vi "Read Shared Variables - SuNLaMP AO v2.vi"(9 "channel errors in (no errors)":errorcluster[](array[cluster])) -> (1 "channel errors out":errorcluster[](array[cluster]), 2 "data":dbl[](array[numeric]), 3 "UUIDs":string[](array[string])=["Flow Rate [g/s]", "Density [g/cm^3]", "Return Filter dP [psid]", "Outlet Filter and Flowmeter dp [psid]", "Cooler dP [psid]", "Cooler CO2 In [F]", "Cooler CO2 Out [F]", "Pump Frequency [%]", "Recirc Valve Open [%]"])   [LabVIEW 2020]
uses:
  <vilib>/ErrorRing/Error Ring.xnode
  <vilib>/Utility/error.llb/Error Cluster From Error Code.vi
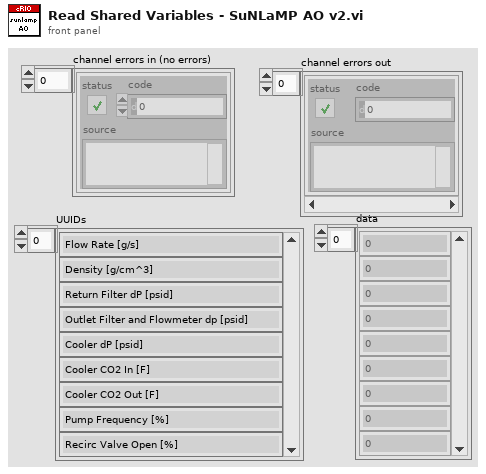
[diagram p1: front panel]
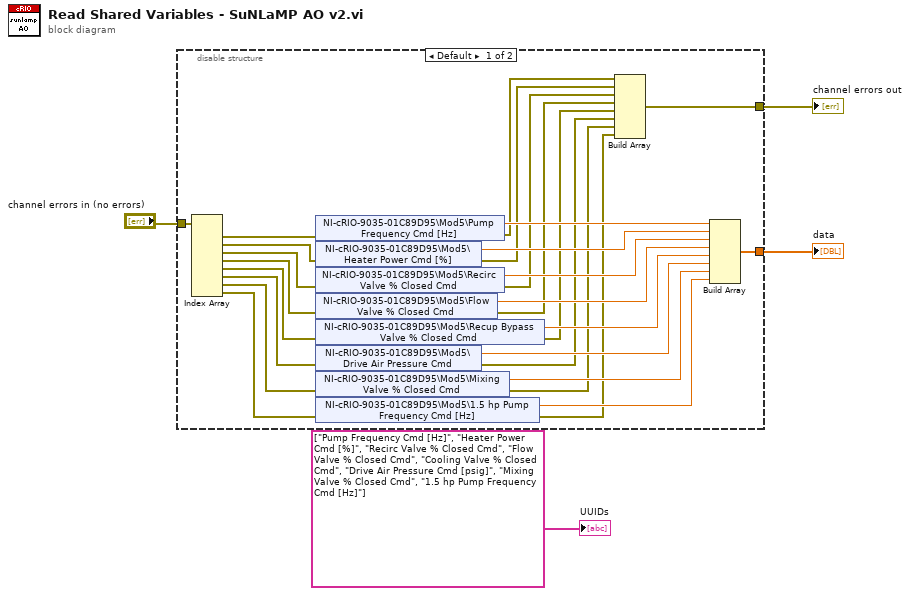
[diagram p0: block diagram]
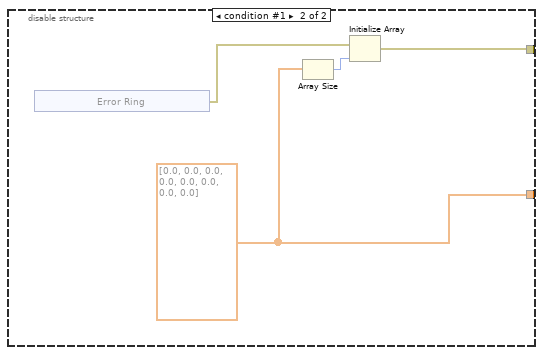
[diagram p2: hidden frame]
diagram:
  n1 = disable-structure shown="Default" {
    disable-tunnel: [w31 w34] -> w4
    disable-tunnel: [w30 w32] -> w2
    disable-tunnel: "channel errors in (no errors)" -> [w29 _]
    frame condition #0 (active) {
      n2 = Index Array(array=w29) -> (element #1=w12:errorcluster, element #2=w11:errorcluster, element #3=w10:errorcluster, element #4=w9:errorcluster, element #5=w8:errorcluster, element #6=w7:errorcluster, element #7=w6:errorcluster, element #8=w5:errorcluster)  [unwired: 8 in]
      n3 = shared-variable "NI-cRIO-9035-01C89D95\\Mod5\\Pump Frequency Cmd [Hz]"(error in=w12) -> (w21:dbl, error out=w13:errorcluster)
      n4 = shared-variable "NI-cRIO-9035-01C89D95\\Mod5\\Heater Power Cmd [%]"(error in=w11) -> (w22:dbl, error out=w14:errorcluster)
      n5 = shared-variable "NI-cRIO-9035-01C89D95\\Mod5\\Recirc Valve % Closed Cmd"(error in=w10) -> (w23:dbl, error out=w15:errorcluster)
      n6 = shared-variable "NI-cRIO-9035-01C89D95\\Mod5\\Flow Valve % Closed Cmd"(error in=w9) -> (w24:dbl, error out=w16:errorcluster)
      n7 = shared-variable "NI-cRIO-9035-01C89D95\\Mod5\\Recup Bypass Valve % Closed Cmd"(error in=w8) -> (w25:dbl, error out=w17:errorcluster)
      n8 = shared-variable "NI-cRIO-9035-01C89D95\\Mod5\\Drive Air Pressure Cmd"(error in=w7) -> (w26:dbl, error out=w18:errorcluster)
      n9 = shared-variable "NI-cRIO-9035-01C89D95\\Mod5\\Mixing Valve % Closed Cmd"(error in=w6) -> (w27:dbl, error out=w19:errorcluster)
      n10 = shared-variable "NI-cRIO-9035-01C89D95\\Mod5\\1.5 hp Pump Frequency Cmd [Hz]"(error in=w5) -> (w28:dbl, error out=w20:errorcluster)
      n11 = Build Array(w13, w14, w15, w16, w17, w18, w19, w20) -> (w30:errorcluster[])
      n12 = Build Array(w21, w22, w23, w24, w25, w26, w27, w28) -> (w31:dbl[])
    }
    frame condition #1 {
      w34 = dbl[] [0.0, 0.0, 0.0, 0.0, 0.0, 0.0, 0.0, 0.0] ("data")
      n13 = xnode "Error Ring"() -> ("error out"=w33:errorcluster)
      n14 = Array Size(array=w34) -> (size(s)=w35:i32)
      n15 = Initialize Array(w33, w35) -> (w32:errorcluster[])
    }
  }
  "data" <- w4
  "channel errors out" <- w2
  "UUIDs" <- string[] ["Pump Frequency Cmd [Hz]", "Heater Power Cmd [%]", "Recirc Valve % Closed Cmd", "Flow Valve % Closed Cmd", "Cooling Valve % Closed Cmd", "Drive Air Pressure Cmd [psig]", "Mixing Valve % Closed Cmd", "1.5 hp Pump Frequency Cmd [Hz]"]
